vi "Pauli-Z_t.vi"(2 "v Ctrl  in":refnum<class "CtrlLine.lvclass">, 7 "QuWire in":refnum<class "QuWire.lvclass">, 13 "^ Ctrl  in":refnum<class "CtrlLine.lvclass">) -> (8 "QuWire out":refnum<class "QuWire.lvclass">)   [LabVIEW 2020]
doc: "Pauli-Z Gate\n\nApplies the Phase Flip. \nLeaves |0> unchanged and maps |1> to -|1>. \nRotates by pi radians around the Z-axis. \n\nMatrix: [[ 1, 0], [ 0, -1]]"
uses:
  QuSim/QuWire/QuWire.lvclass
  QuSim/QuWire/CtrlLine/CtrlLine.lvclass
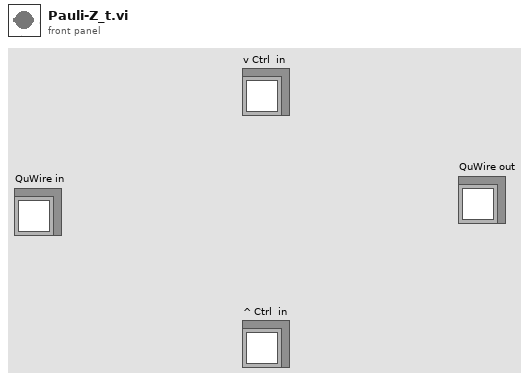
[diagram p1: front panel]
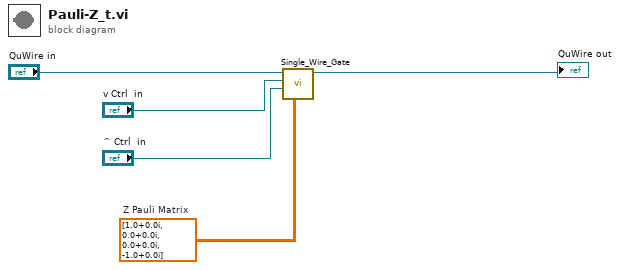
[diagram p0: block diagram]
diagram:
  w1 = cdb[][] [[1.0+0.0i, 0.0+0.0i], [0.0+0.0i, -1.0+0.0i]]  # Z Pauli Matrix
  n1 = call "Single_Wire_Gate.vi"("2x2 Unitary Matrix"=w1, "d CtrlLine in"="^ Ctrl  in", "u CtrlLine in"="v Ctrl  in", "QuWire in"="QuWire in") -> ("QuWire out"=→"QuWire out":refnum<class "QuWire.lvclass">)  [unwired: 6 in, 1 out]
